vi "Calculate Elapsed Time.vi"(10 "StartTime":string, 11 "time string":string) -> (3 "Elapsed Seconds":string)   [LabVIEW 2020, in "WritingDataFile.lvlib"]
uses:
  WritingDataFile.lvlib
panel:
  out "Time Difference (HH:MM:SS)":dbl format="%<%H:%M:%S>t"
  out "Time Difference (Seconds)":dbl
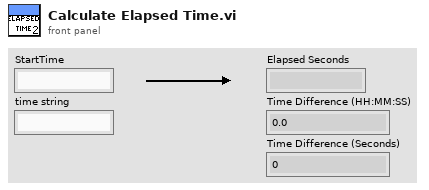
[diagram p1: front panel]
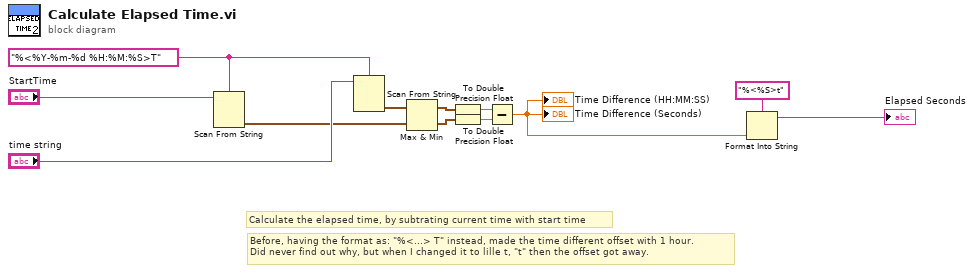
[diagram p0: block diagram]
diagram:
  w12 = "%<%Y-%m-%d %H:%M:%S>T" ("format string")
  # "Before, having the format as: \"%<...> T\" instead, made the time different offset with 1 hour. \nDid never find out why, but when I changed it to lille t, \"t\" then the offset got away."
  # "Calculate the elapsed time, by subtrating current time with start time"
  n1 = Scan From String(format string=w12, input string="StartTime") -> (output 1=w2:timestamp)  [unwired: 3 in, 3 out]
  n2 = Scan From String(format string=w12, input string="time string") -> (output 1=w1:timestamp)  [unwired: 3 in, 3 out]
  n3 = Max & Min(x=w1, y=w2) -> (max(x,y)=w3:timestamp, min(x,y)=w4:timestamp)
  n4 = To Double Precision Float(number=w3) -> (double precision float=w5:dbl)
  n5 = To Double Precision Float(number=w4) -> (double precision float=w6:dbl)
  n6 = Subtract(x=w5, y=w6) -> (x-y=w8:dbl)
  "Time Difference (Seconds)" <- w8
  "Time Difference (HH:MM:SS)" <- w8
  n7 = Format Into String(format string="%<%S>t", w8) -> (resulting string=→"Elapsed Seconds":string)  [unwired: 2 in, 1 out]
